vi "Manage Transition.vi"(6 "Force transition":bool, 11 "Game Board in":refnum<class "Game Board.lvclass">) -> (3 "Game Board out":refnum<class "Game Board.lvclass">, 4 "Exit?":bool, 5 "State out":T1=enum."Playing")   [LabVIEW 2024, in "Game Board.lvclass"]
doc: "MIT Licence\nCopyright (c) 2024 David Grollier"
uses:
  Game Board.lvclass
  Type Def/State Main.ctl
  Game Board.lvclass/Game Board.ctl
  <vilib>/ptbypt/NI_PtbyPt.lvlib
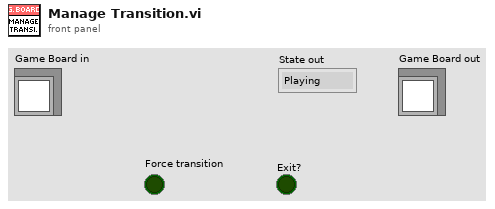
[diagram p1: front panel]
types:
  T1 = typedef "State Main.ctl" = enum16{"init", "Timer", "Playing"}
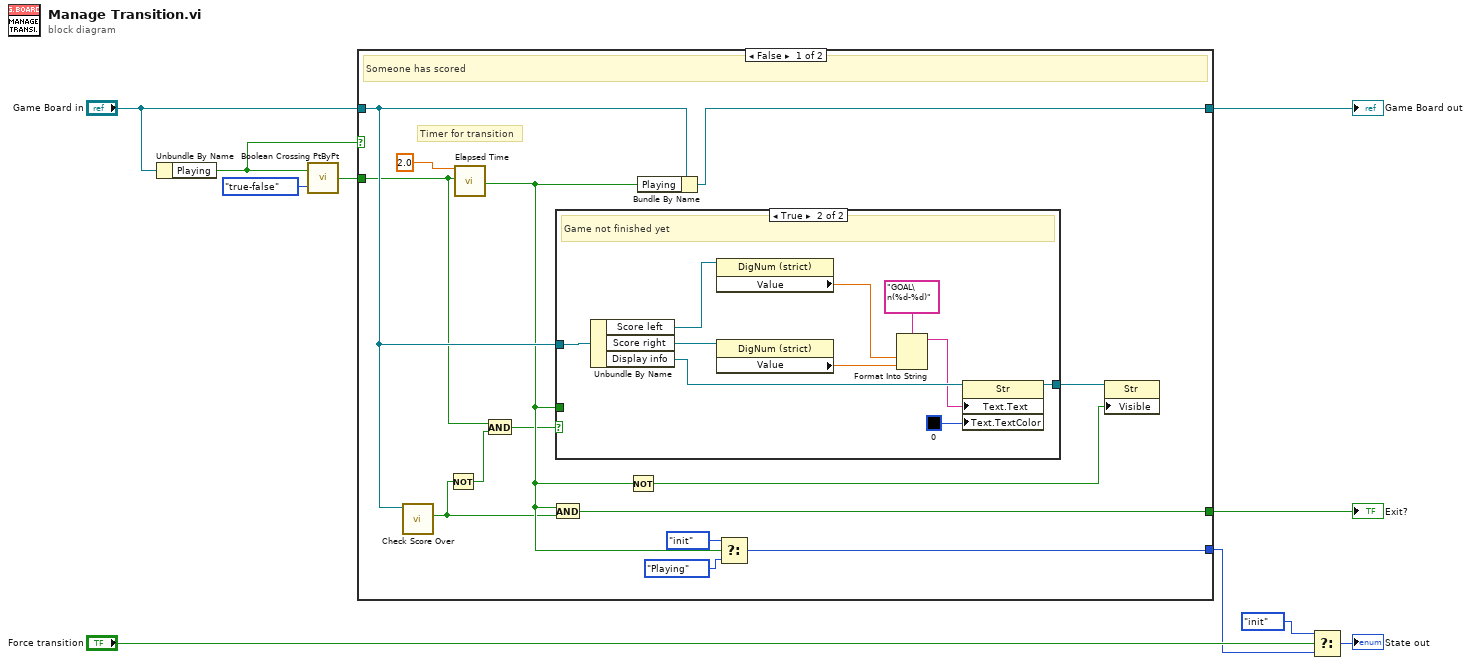
[diagram p0: block diagram]
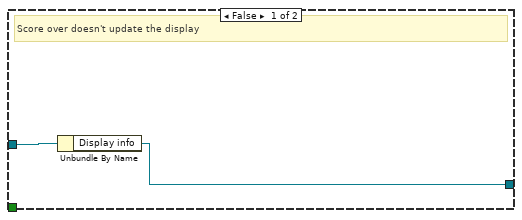
[diagram p2: hidden frame]
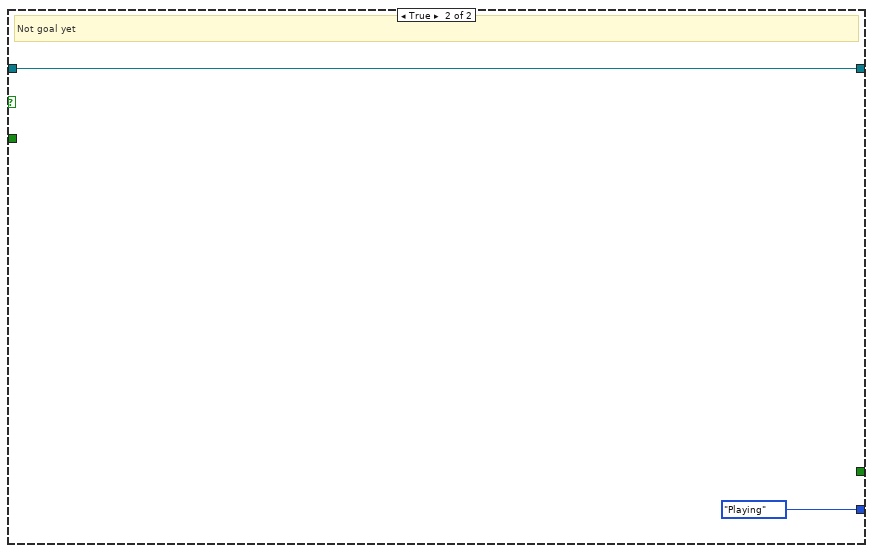
[diagram p3: hidden frame]
diagram:
  n1 = Unbundle By Name("Game Board in") -> ("Playing"=w5:bool)
  n2 = call <vilib>:"Boolean Crossing PtByPt.vi"("direction"=enum16{"either", "false-true", "true-false"}."true-false", "input"=w5) -> ("crossing"=w7:bool)  [unwired: 1 in]
  n3 = case shown="False" w5 {
    tunnel: w7 -> [w13 _]
    tunnel: "Game Board in" -> [w22 w38]
    tunnel: [w23 w38] -> w4
    tunnel: [w11 State_Main."Playing" ("State out")] -> w3
    tunnel: [w19 _] -> w1
    frame False {
      # "Timer for transition"
      # "Someone has scored"
      n4 = call "Check Score Over.vi"("Game Board in"=w22) -> ("Score over?"=w15:bool)  [unwired: 10 in]
      n5 = Not(x=w15) -> (.not. x?=w14:bool)
      n6 = call "Elapsed Time"("Time Target (s)"=2.0, "Reset"=w13) -> ("Time has Elapsed"=w17:bool)  [unwired: 10 in, 7 out]
      n7 = And(x=w13, y=w14) -> (x .and. y?=w12:bool)
      n8 = And(x=w17, y=w15) -> (x .and. y?=w19:bool)
      n9 = case shown="True" w12 {
        tunnel: w17 -> [_ _]
        tunnel: w22 -> [w26 w34]
        tunnel: [w25 w27] -> w18
        frame False {
          # "Score over doesn't update the display"
          n10 = Unbundle By Name(w26) -> ("Display info"=w25:refnum<vi>)
        }
        frame True {
          # "Game not finished yet"
          n11 = Unbundle By Name(w34) -> ("Score left"=w31:refnum<vi>, "Score right"=w32:refnum<vi>, "Display info"=w35:refnum<vi>)
          n12 = property class="DigNum (strict)"(reference=w31) -> ("Value"=w29:dbl)  [unwired: 1 in, 2 out]
          n13 = property class="DigNum (strict)"(reference=w32) -> ("Value"=w30:dbl)  [unwired: 1 in, 2 out]
          n14 = Format Into String(format string="GOAL\n(%d-%d)", w29, w30) -> (resulting string=w28:string)  [unwired: 2 in, 1 out]
          n15 = property class="Str"(reference=w35, "Text.Text"=w28, "Text.TextColor"=u32 0 ("Text.Text Colors:Text Color")) -> (reference out=w27:refnum<vi>)  [unwired: 1 in, 1 out]
        }
      }
      n16 = Not(x=w17) -> (.not. x?=w16:bool)
      n17 = Bundle By Name(cluster=w22, "Playing"=w17) -> (w23:refnum<class "Game Board.lvclass">)
      n18 = Select(t=State_Main."init" ("f"), s=w17, f=State_Main."Playing" ("State out")) -> (s? t:f=w11:T1)
      n19 = property class="Str"(reference=w18, "Visible"=w16) -> ()  [unwired: 1 in, 2 out]
    }
    frame True {
      # "Not goal yet"
    }
  }
  "Game Board out" <- w4
  "Exit?" <- w1
  n20 = Select(t=State_Main."init" ("State out"), s="Force transition", f=w3) -> (s? t:f=→"State out":T1)
